vi "Arduinopractice.vi"() -> ()   [LabVIEW 2013]
uses:
  <vilib>/LabVIEW Interface for Arduino/Type Defs/Pin Mode.ctl
  <vilib>/LabVIEW Interface for Arduino/LabVIEW Interface for Arduino.lvlib
panel:
  out "Boolean 2":bool
  in  "Digital I/O Pin":u8=13
  in  "Boolean":bool
  in  "stop":bool
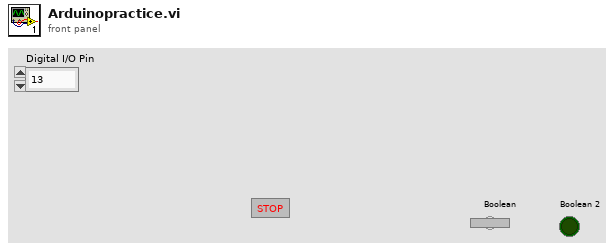
[diagram p1: front panel]
types:
  T1 = typedef "LabVIEW Interface for Arduino.lvlib/Pin Mode.ctl" = enum8{"Input", "Output"}
  T2 = typedef "LabVIEW Interface for Arduino.lvlib/Arduino Resource.ctl" = cluster{"VISA resource":refnum<visa-resource-name>, "Board Type":T3, "Connection Type":enum8{"USB / Serial"}, "Bytes Per Packet (15)":u8}
  T3 = typedef "LabVIEW Interface for Arduino.lvlib/Board Type.ctl" = enum16{"Uno", "Dimuelanove w/Atmega 328", "Mega 2560"}
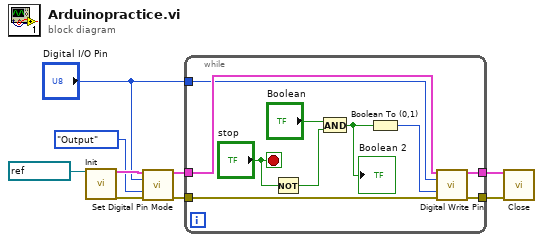
[diagram p0: block diagram]
diagram:
  n1 = call <vilib>:"Init.vi"("VISA resource"=refnum<visa-resource-name> "COM3") -> ("Arduino Resource"=w9:T2, "error out"=w8:errorcluster)  [unwired: 17 in]
  n2 = call <vilib>:"Set Digital Pin Mode.vi"("Arduino Resource"=w9, "Digital I/O Pin"="Digital I/O Pin", "Pin Mode (Input)"=Pin_Mode."Output", "error in"=w8) -> ("Arduino Resource"=w6:T2, "error out"=w5:errorcluster)  [unwired: 10 in]
  n3 = while {
    tunnel: w6 -> [w19]
    tunnel: w5 -> [w18]
    tunnel: [w17] -> w4
    tunnel: [w16] -> w3
    tunnel: "Digital I/O Pin" -> [w15]
    stop <- "stop" stop-if-true
    n4 = Not(x="stop") -> (.not. x?=w12:bool)
    n5 = And(x="Boolean", y=w12) -> (x .and. y?=w10:bool)
    "Boolean 2" <- w10
    n6 = Boolean To (0,1)(Boolean=w10) -> (0, 1=w14:i16)
    n7 = call <vilib>:"Digital Write Pin.vi"("Arduino Resource"=w19, "Digital I/O Pin (0)"=w15, "Value (0)"=w14, "error in"=w18) -> ("Arduino Resource"=w16:T2, "error out"=w17:errorcluster)  [unwired: 10 in]
  }
  n8 = call <vilib>:"Close.vi"("Arduino Resource"=w3, "error in"=w4) -> ()  [unwired: 13 in, 1 out]
